vi "Scan Cluster.vi"(8 "Error In":errorcluster, 11 "Value":variant) -> (0 "Error Out":errorcluster, 2 "Changed":bool[](array[boolean]), 3 "Control names":string[](array[string]))   [LabVIEW 2019]
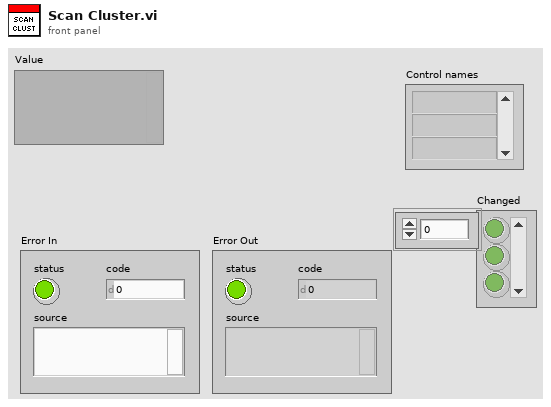
[diagram p1: front panel]
types:
  T1 = typedef "Type Descriptor Enumeration__ogtk.ctl" = enum8{"<Null>", "I8", "I16", "I32", "I64", "U8", "U16", "U32", "U64", "SGL", "DBL", "EXT", "CSG", "CDB", "CXT", "0x0F", "0x10", "0x11", "0x12", "0x13", "0x14", "Enum U8", "Enum U16", "Enum U32", "Enum U64", "SGL PQ", "DBL PQ", "EXT PQ", "CSG PQ", "CDB PQ", "CXT PQ", "0x1F", "0x20", "Boolean", "0x22", "0x23", "0x24", "0x25", "0x26", "0x27", "0x28", "0x29", "0x2A", "0x2B", "0x2C", "0x2D", "0x2E", "0x2F", "String", "0x31", "Path", "Pict", "0x34", "0x35", "0x36", "DAQ", "0x38", "0x39", "0x3A", "0x3B", "0x3C", "0x3D", "0x3E", "0x3F", "Array", "0x41", "0x42", "0x43", "0x44", "0x45", "0x46", "0x47", "0x48", "0x49", "0x4A", "0x4B", "0x4C", "0x4D", "0x4E", "0x4F", "Cluster", "0x51", "0x52", "Variant", "Waveform", "0x55", "0x56", "0x57", "0x58", "0x59", "0x5A", "0x5B", "0x5C", "0x5D", "0x5E", "Fixed Point", "0x60", "0x61", "0x62", "0x63", "0x64", "0x65", "0x66", "0x67", "0x68", "0x69", "0x6A", "0x6B", "0x6C", "0x6D", "0x6E", "0x6F", "Refnum", "0x71", "0x72", "Set Collection", "Map Collection"}
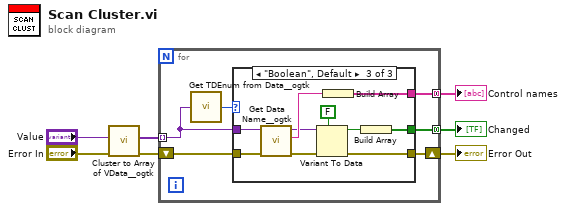
[diagram p0: block diagram]
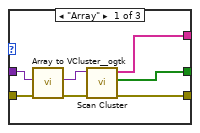
[diagram p2: hidden frame]
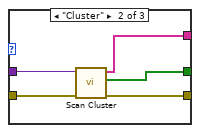
[diagram p3: hidden frame]
diagram:
  n1 = call <userlib>:"Cluster to Array of VData__ogtk.vi"("error in (no error)"="Error In", "Cluster"="Value") -> ("error out"=w3:errorcluster, "Array of VData"=w7:variant[])  [unwired: 8 in]
  n2 = for {
    tunnel: w7 -> [w12] mode=indexing
    tunnel: [w11] -> w5 mode=concatenating
    tunnel: [w10] -> w6 mode=concatenating
    shift-right: [w8] -> w2
    shift-left: w3 -> [w9]
    n3 = call <userlib>:"Get TDEnum from Data__ogtk.vi"("Data"=w12) -> ("Type Descriptor Enumeration"=w13:T1)  [unwired: 4 in]
    n4 = case shown="\"Boolean\", Default" w13 {
      tunnel: w12 -> [w20 w21 w35]
      tunnel: [w18 w22 w31] -> w11
      tunnel: [w17 w23 w30] -> w10
      tunnel: w9 -> [w16 w25 w29]
      tunnel: [w14 w24 w26] -> w8
      frame "Array" {
        n5 = call <userlib>:"Array to VCluster__ogtk.vi"("error in (no error)"=w16, "Array"=w20) -> ("error out"=w15:errorcluster, "VCluster"=w19:variant)  [unwired: 8 in]
        n6 = call "Scan Cluster.vi"("Error In"=w15, "Value"=w19) -> ("Error Out"=w14:errorcluster, "Changed"=w17:bool[], "Control names"=w18:string[])  [unwired: 7 in]
      }
      frame "Cluster" {
        n7 = call "Scan Cluster.vi"("Error In"=w25, "Value"=w21) -> ("Error Out"=w24:errorcluster, "Changed"=w23:bool[], "Control names"=w22:string[])  [unwired: 7 in]
      }
      frame "Boolean", Default {
        n8 = call <userlib>:"Get Data Name__ogtk.vi"("error in (no error)"=w29, "Data"=w35) -> ("error out"=w27:errorcluster, "Data Name"=w33:string, "Data dup"=w28:variant)  [unwired: 7 in]
        n9 = Variant To Data(error in=w27, type=FALSE, Variant=w28) -> (data=w32:bool, error out=w26:errorcluster)
        n10 = Build Array(w33) -> (w31:string[])
        n11 = Build Array(w32) -> (w30:bool[])
      }
    }
  }
  "Control names" <- w5
  "Changed" <- w6
  "Error Out" <- w2
